vi "Expand shift register.vi"(7 "Add after register":i32, 8 "error in (no error)":errorcluster, 9 "New Left register count":i32, 10 "Outer Terminal Sources":refnum<vi>[](array[refnum]), 11 "Shift Register":refnum<vi>) -> (0 "error out":errorcluster, 1 "Inner Terminals":refnum<vi>[](array[refnum]), 2 "Outer Terminals":refnum<vi>[](array[refnum]), 3 "New Shift Registers":refnum<vi>[](array[refnum]))   [LabVIEW 2012, in "Scripting Tools.lvlib"]
doc: "Adds new left elements to <b>Shift Register</b>, optionally wiring up the new elements inner and out terminals"
uses:
  Scripting Tools.lvlib
panel:
  in  "Inner Terminal sinks":refnum<vi>[](array[refnum])
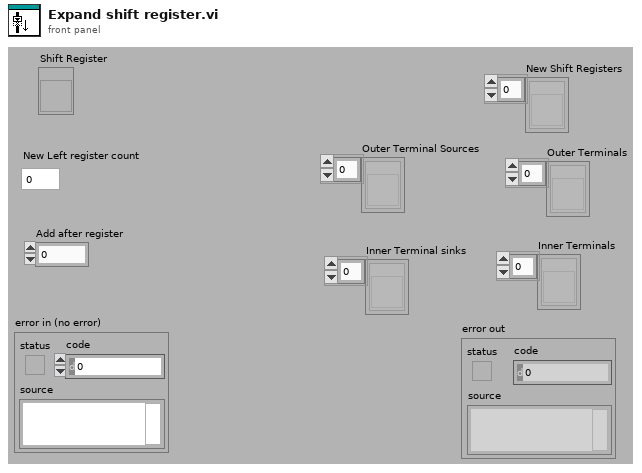
[diagram p1: front panel]
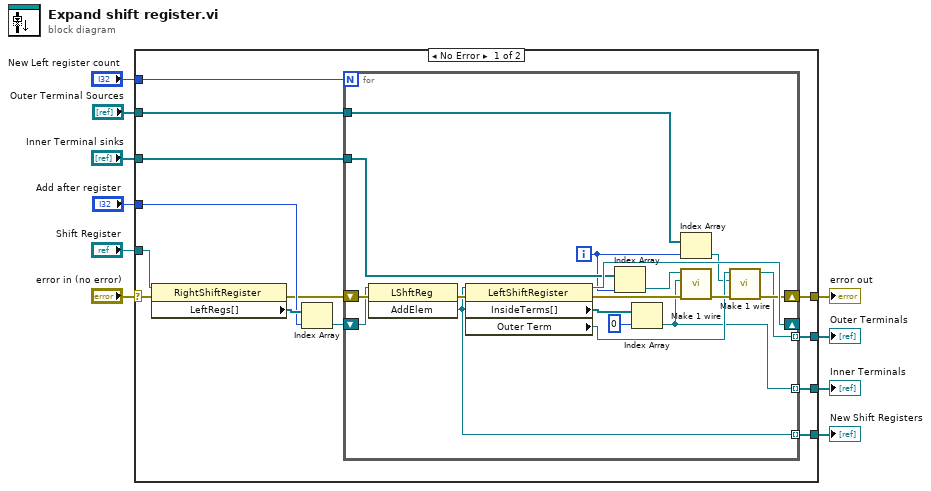
[diagram p0: block diagram]
diagram:
  n1 = case shown="No Error" "error in (no error)" {
    selector: "error in (no error)" -> [w22 w42]
    tunnel: "Shift Register" -> [w23 _]
    tunnel: "Add after register" -> [w20 _]
    tunnel: "New Left register count" -> [w18 _]
    tunnel: "Inner Terminal sinks" -> [w16 _]
    tunnel: "Outer Terminal Sources" -> [w15 _]
    tunnel: [w14 _] -> w4
    tunnel: [w13 _] -> w3
    tunnel: [w12 w42] -> w2
    tunnel: [w11 _] -> w1
    frame No Error {
      n2 = property class="RightShiftRegister"(reference=w23, error in=w22) -> (error out=w17:errorcluster, "LeftRegs[]"=w21:refnum<vi>[])  [unwired: 1 out]
      n3 = Index Array(array=w21, index=w20) -> (element=w19:refnum<vi>)
      n4 = for {
        N: w18 -> [_]
        shift-right: [w38] -> _
        shift-left: w19 -> [w40]
        shift-right: [w32] -> w12
        shift-left: w17 -> [w41]
        tunnel: [w31] -> w14 mode=indexing
        tunnel: [w30] -> w13 mode=indexing
        tunnel: w16 -> [w29]
        tunnel: w15 -> [w28]
        tunnel: [w27] -> w11 mode=indexing
        i -> [w24]
        n5 = invoke class="LShftReg" method="AddElem"(reference=w40, error in=w41) -> (error out=w39:errorcluster, "AddElem"=w27:refnum<vi>)  [unwired: 1 in, 1 out]
        n6 = property class="LeftShiftRegister"(reference=w27, error in=w39) -> (reference out=w38:refnum<vi>, error out=w35:errorcluster, "InsideTerms[]"=w37:refnum<vi>[], "Outer Term"=w33:refnum<vi>)
        n7 = Index Array(array=w29, index=w24) -> (element=w26:refnum<vi>)
        n8 = Index Array(array=w37, index=0) -> (element=w30:refnum<vi>)
        n9 = Index Array(array=w28, index=w24) -> (element=w25:refnum<vi>)
        n10 = call "Make 1 wire.vi"("error in"=w35, "Wire Terminal 2"=w30, "Wire Terminal 1"=w26) -> ("error out"=w34:errorcluster)  [unwired: 8 out]
        n11 = call "Make 1 wire.vi"("error in"=w34, "Wire Terminal 2"=w25, "Wire Terminal 1"=w33) -> ("error out"=w32:errorcluster, "Wire Sink Terminal Out"=w31:refnum<vi>)  [unwired: 7 out]
      }
    }
    frame Error {
    }
  }
  "error out" <- w2
  "Outer Terminals" <- w4
  "Inner Terminals" <- w3
  "New Shift Registers" <- w1
